vi "TcA07-005_InterfaceSupportMethods.vi"(1 "Input buffer":T3="1", 3 "Invocation info":T2, 5 "error in (no error)":errorcluster, 6 "Add log to result?":bool) -> (16 "Test Data":T1 {"Numeric Measurement" format="%.2f"}, 19 "error out":errorcluster)   [LabVIEW 2009]
doc: "Test case template."
uses:
  Shared/Support_InputBuffer.ctl
  Shared/Support_InvocationInfo.ctl
  Shared/Support_TestData.ctl
  <vilib>/addons/_AddQ/G#Object/G#Object.lvclass
  TestClasses/G#BaseClass2_class/interfaces/G#BaseClass2_IG#BaseInterface/G#BaseClass2_IG#BaseInterface.lvclass
  <vilib>/addons/_AddQ/G#Interface/G#Interface.lvclass
  TestClasses/G#BaseClass1_class/interfaces/G#BaseClass1_IG#BaseInterface/G#BaseClass1_IG#BaseInterface.lvclass
  TestClasses/G#SubClass2_class/G#SubClass2.lvclass
  TestClasses/G#SubClass1_class/G#SubClass1.lvclass
panel:
  in  "Test name":string="TcA07-005 Interface Support Methods"
  out "Test result":bool
  out "Result":string
  # "Verify that the support methods works as expected."
  # "Sub test case"
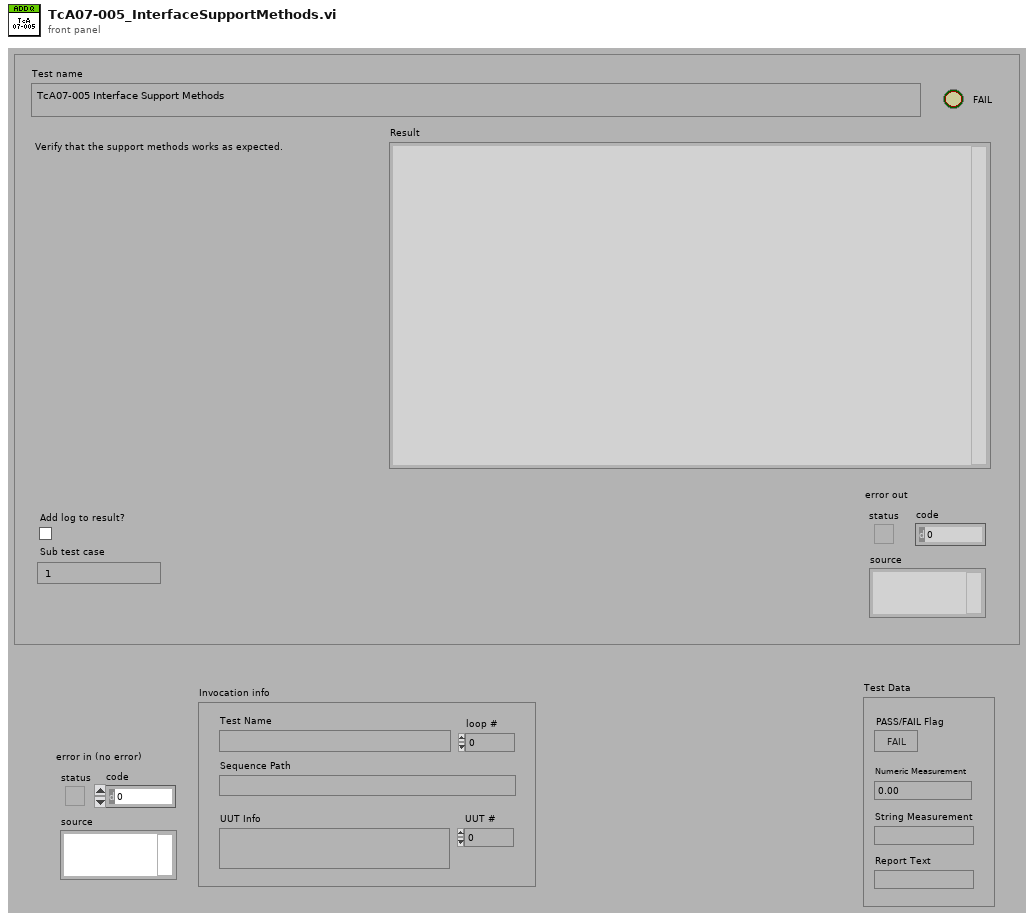
[diagram p1: front panel]
types:
  T1 = typedef "Support_TestData.ctl" = cluster{"PASS/FAIL Flag":bool, "Numeric Measurement":dbl, "String Measurement":string, "Report Text":string}
  T2 = typedef "Support_InvocationInfo.ctl" = cluster{"UUT #":i32, "loop #":i32, "UUT Info":string, "Test Name":string, "Sequence Path":path}
  T3 = typedef "Support_InputBuffer.ctl" = string
  T4 = typedef "Support_ResultType.ctl" = cluster{"Pass":bool, "Comment":string, "MeasurementValue":dbl}
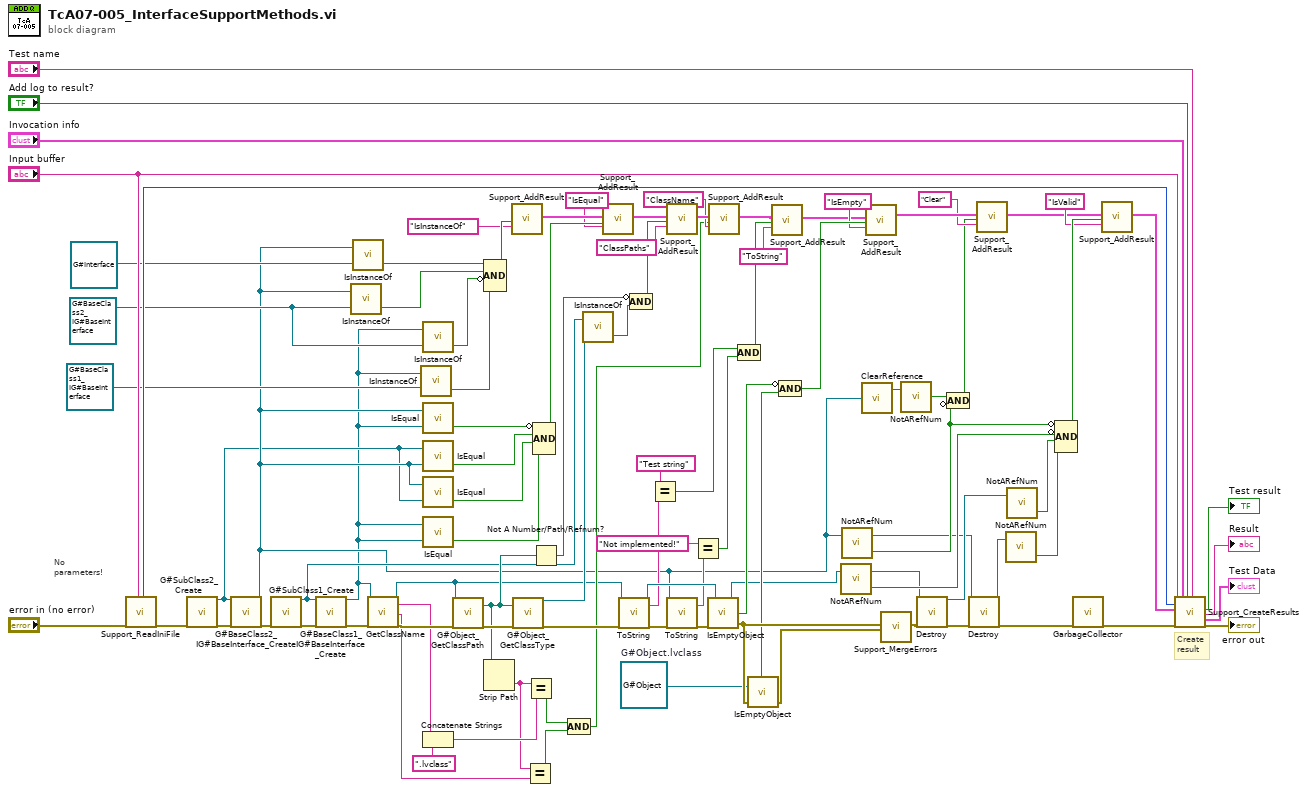
[diagram p0: block diagram]
diagram:
  w11 = refnum<class "G#BaseClass2_IG#BaseInterface.lvclass"> refnum ("reference out")
  w18 = refnum<class "G#Object.lvclass"> refnum  # G#Object.lvclass
  # "No\nparameters!"
  # "Create\nresult"
  n1 = call "Support_ReadIniFile.vi"("error in (no error)"="error in (no error)", "Sub test case"="Input buffer") -> ("Timer start"=w89:u32, "error out"=w87:errorcluster)  [unwired: 10 in, 6 out]
  n2 = call "G#SubClass2_Create.vi"("error in (no error)"=w87) -> ("reference out"=w7:refnum<class "G#SubClass2.lvclass">, "error out"=w17:errorcluster)  [unwired: 17 in]
  n3 = call "G#BaseClass2_IG#BaseInterface_Create.vi"("reference in"=w7, "error in (no error)"=w17) -> ("reference out"=w8:refnum<class "G#BaseClass2_IG#BaseInterface.lvclass">, "error out"=w16:errorcluster)  [unwired: 16 in]
  n4 = call "G#SubClass1_Create.vi"("error in (no error)"=w16) -> ("reference out"=w13:refnum<class "G#SubClass1.lvclass">, "error out"=w15:errorcluster)  [unwired: 16 in, 1 out]
  n5 = call "G#BaseClass1_IG#BaseInterface_Create.vi"("reference in"=w13, "error in (no error)"=w15) -> ("reference out"=w5:refnum<class "G#BaseClass1_IG#BaseInterface.lvclass">, "error out"=w14:errorcluster)  [unwired: 16 in]
  n6 = call-dynamic "IsInstanceOf.vi"("is object instance of"=w11, "reference in"=w8) -> ("is instance of"=w83:bool)  [unwired: 1 out]
  n7 = call-dynamic "IsInstanceOf.vi"("is object instance of"=refnum<class "G#Interface.lvclass"> refnum ("reference in"), "reference in"=w8) -> ("is instance of"=w84:bool)  [unwired: 1 out]
  n8 = call-dynamic "GetClassName.vi"("reference in"=w5, "error in (no error)"=w14) -> ("reference out"=w9:refnum<class "G#BaseClass1_IG#BaseInterface.lvclass">, "class name"=w47:string, "full class name"=w43:string, "error out"=w57:errorcluster)  [unwired: 13 in, 1 out]
  n9 = call-dynamic "IsInstanceOf.vi"("is object instance of"=refnum<class "G#BaseClass1_IG#BaseInterface.lvclass"> refnum ("reference out"), "reference in"=w5) -> ("is instance of"=w81:bool)  [unwired: 1 out]
  n10 = call-dynamic "IsInstanceOf.vi"("is object instance of"=w11, "reference in"=w5) -> ("is instance of"=w82:bool)  [unwired: 1 out]
  n11 = call-dynamic "IsEqual.vi"("is equal to"=w5, "reference in"=w8) -> ("is equal?"=w62:bool)  [unwired: 1 out]
  n12 = call-dynamic "IsEqual.vi"("is equal to"=w8, "reference in"=w7) -> ("is equal"=w61:bool)  [unwired: 1 out]
  n13 = call-dynamic "IsEqual.vi"("is equal to"=w7, "reference in"=w8) -> ("is equal?"=w6:bool)  [unwired: 1 out]
  n14 = call-dynamic "IsEqual.vi"("is equal to"=w5, "reference in"=w5) -> ("is equal?"=w4:bool)  [unwired: 1 out]
  n15 = Concatenate Strings(w47, ".lvclass" ("string")) -> (w45:string)
  n16 = call-dynamic "G#Object_GetClassPath.vi"("reference in"=w9, "error in (no error)"=w57) -> ("class path"=w48:path, "error out"=w56:errorcluster)  [unwired: 15 in, 1 out]
  n17 = Compound Arithmetic op=AND(w84, w83, invert w82, w81) -> (w80:bool)
  n18 = Strip Path(path=w48) -> (name=w44:string)  [unwired: 1 out]
  n19 = call "Support_AddResult.vi"("Pass"=w80, "Comment"="IsInstanceOf") -> ("Results out"=w60:T4[])  [unwired: 17 in]
  n20 = call <vilib>:"G#Object_GetClassType.vi"("class path"=w48, "error in (no error)"=w56) -> ("reference out"=w55:refnum<class "G#Object.lvclass">, "error out"=w54:errorcluster)  [unwired: 16 in]
  n21 = Equal?(x=w44, y=w43) -> (x = y?=w41:bool)
  n22 = Equal?(x=w44, y=w45) -> (x = y?=w42:bool)
  n23 = Not A Number/Path/Refnum?(number/path/refnum=w48) -> (NaN/Path/Refnum?=w50:bool)
  n24 = Compound Arithmetic op=AND(invert w62, w61, w6, w4) -> (w59:bool)
  n25 = Compound Arithmetic op=AND(w42, w41) -> (w19:bool)
  n26 = call-dynamic "IsInstanceOf.vi"("is object instance of"=w55, "reference in"=w13) -> ("is instance of"=w51:bool)  [unwired: 1 out]
  n27 = call "Support_AddResult.vi"("Results in"=w60, "Pass"=w59, "Comment"="IsEqual") -> ("Results out"=w52:T4[])  [unwired: 16 in]
  n28 = call-dynamic "ToString.vi"("reference in"=w9, "error in (no error)"=w54) -> ("reference out"=w53:refnum<class "G#BaseClass1_IG#BaseInterface.lvclass">, "string"=w38:string, "error out"=w37:errorcluster)  [unwired: 15 in]
  n29 = Compound Arithmetic op=AND(invert w50, w51) -> (w21:bool)
  n30 = Equal?(x="Test string", y=w38) -> (x = y?=w33:bool)
  n31 = call "Support_AddResult.vi"("Results in"=w52, "Pass"=w21, "Comment"="ClassPaths") -> ("Results out"=w22:T4[])  [unwired: 16 in]
  n32 = call-dynamic "ToString.vi"("reference in"=w8, "error in (no error)"=w37) -> ("string"=w35:string, "error out"=w36:errorcluster)  [unwired: 15 in, 1 out]
  n33 = Equal?(x="Not implemented!", y=w35) -> (x = y?=w32:bool)
  n34 = call-dynamic "IsEmptyObject.vi"("error in (no error)"=w36, "reference in"=w53) -> ("error out"=w71:errorcluster, "is empty?"=w69:bool, "reference out"=w3:refnum<class "G#BaseClass1_IG#BaseInterface.lvclass">)  [unwired: 1 in]
  n35 = call "Support_AddResult.vi"("Results in"=w22, "Pass"=w19, "Comment"="ClassName") -> ("Results out"=w23:T4[])  [unwired: 16 in]
  n36 = Compound Arithmetic op=AND(w33, w32) -> (w31:bool)
  n37 = call-dynamic "IsEmptyObject.vi"("error in (no error)"=w71, "reference in"=w18) -> ("error out"=w70:errorcluster, "is empty?"=w68:bool)  [unwired: 1 in, 1 out]
  n38 = call "Support_AddResult.vi"("Results in"=w23, "Pass"=w31, "Comment"="ToString") -> ("Results out"=w40:T4[])  [unwired: 16 in]
  n39 = Compound Arithmetic op=AND(invert w69, w68) -> (w67:bool)
  n40 = call-dynamic "NotARefNum.vi"("reference in"=w3) -> ("not a refnum?"=w76:bool, "reference out"=w2:refnum<class "G#BaseClass1_IG#BaseInterface.lvclass">)  [unwired: 1 in]
  n41 = call-dynamic "NotARefNum.vi"("reference in"=w8) -> ("not a refnum?"=w26:bool, "reference out"=w1:refnum<class "G#BaseClass2_IG#BaseInterface.lvclass">)  [unwired: 1 in]
  n42 = call-dynamic "ClearReference.vi"("reference in"=w8) -> ("reference out"=w72:refnum<class "G#BaseClass2_IG#BaseInterface.lvclass">)
  n43 = call "Support_AddResult.vi"("Results in"=w40, "Pass"=w67, "Comment"="IsEmpty") -> ("Results out"=w29:T4[])  [unwired: 16 in]
  n44 = call "Support_MergeErrors.vi"("error in 1"=w71, "error in 2"=w70) -> ("error out"=w73:errorcluster)  [unwired: 16 in, 1 out]
  n45 = call-dynamic "NotARefNum.vi"("reference in"=w72) -> ("not a refnum?"=w25:bool)  [unwired: 1 in, 1 out]
  n46 = call-dynamic "Destroy.vi"("reference in"=w2, "error in (no error)"=w73) -> ("reference out"=w78:refnum<class "G#BaseClass1_IG#BaseInterface.lvclass">, "error out"=w85:errorcluster)  [unwired: 16 in]
  n47 = Compound Arithmetic op=AND(w25, invert w26) -> (w24:bool)
  n48 = call-dynamic "Destroy.vi"("reference in"=w1, "error in (no error)"=w85) -> ("reference out"=w77:refnum<class "G#BaseClass2_IG#BaseInterface.lvclass">, "error out"=w86:errorcluster)  [unwired: 16 in]
  n49 = call "Support_AddResult.vi"("Results in"=w29, "Pass"=w24, "Comment"="Clear") -> ("Results out"=w28:T4[])  [unwired: 16 in]
  n50 = call-dynamic "NotARefNum.vi"("reference in"=w77) -> ("not a refnum?"=w74:bool)  [unwired: 1 in, 1 out]
  n51 = call-dynamic "NotARefNum.vi"("reference in"=w78) -> ("not a refnum?"=w75:bool)  [unwired: 1 in, 1 out]
  n52 = Compound Arithmetic op=AND(invert w26, invert w76, w75, w74) -> (w66:bool)
  n53 = call <vilib>:"GarbageCollector.vi"("error in (no error)"=w86) -> ("error out"=w88:errorcluster)  [unwired: 16 in, 2 out]
  n54 = call "Support_AddResult.vi"("Results in"=w28, "Pass"=w66, "Comment"="IsValid") -> ("Results out"=w65:T4[])  [unwired: 16 in]
  n55 = call "Support_CreateResults.vi"("Sub test case"="Input buffer", "Timer start"=w89, "Results"=w65, "error in (no error)"=w88, "Invocation info"="Invocation info", "Add log to result?"="Add log to result?", "Test name"="Test name") -> ("Pass/fail flag"=→"Test result":bool, "Result"=→"Result":string, "Test Data"=→"Test Data":T1, "error out"=→"error out":errorcluster)  [unwired: 9 in]
